vi "Canny Edge Detection.vi"(4 "Threshold 2":dbl=100.0, 6 "Threshold 1":dbl=50.0, 7 "Aperture Size":T1, 8 "error in (no error)":errorcluster, 10 "Canny Edge Result in":T2, 11 "Greyscale Image-Source in":T2) -> (0 "error out":errorcluster, 3 "Canny Edge":T2)   [LabVIEW 2020, in "image.lvlib"]
doc: "Apply the Canny Edge Detetction operation to the source image."
uses:
  image.lvlib
  Greyscale Image.ctl
  Canny Aperture Size.ctl
  common/common.lvlib
  common/bin/gartoolkit_32-1.dll
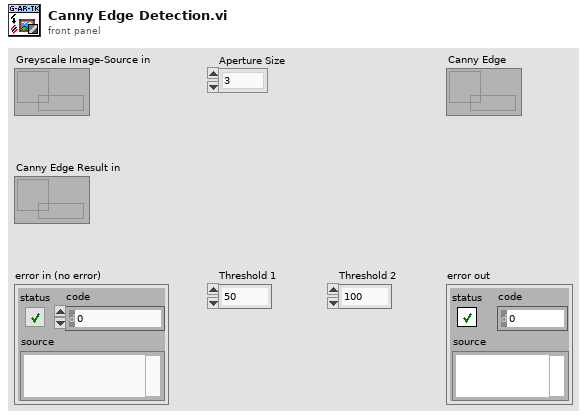
[diagram p1: front panel]
types:
  T1 = typedef "image.lvlib/Canny Aperture Size.ctl" = enum16{"3", "5", "7"}
  T2 = typedef "image.lvlib/Greyscale Image.ctl" = refnum<data-value>
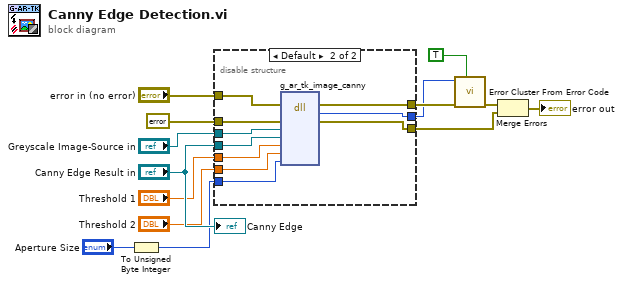
[diagram p0: block diagram]
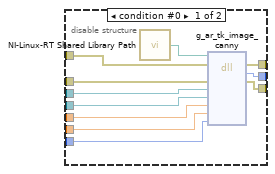
[diagram p2: hidden frame]
diagram:
  n1 = To Unsigned Byte Integer(number="Aperture Size") -> (unsigned 8bit integer=w5:u8)
  n2 = disable-structure shown="Default" {
    disable-tunnel: "error in (no error)" -> [w25 w35]
    disable-tunnel: errorcluster {"status"=FALSE, "code"=0, "source"=""} ("error constant") -> [w24 w34]
    disable-tunnel: "Greyscale Image-Source in" -> [w23 w33]
    disable-tunnel: "Canny Edge Result in" -> [w22 w32]
    disable-tunnel: "Threshold 1" -> [w21 w31]
    disable-tunnel: "Threshold 2" -> [w20 w30]
    disable-tunnel: w5 -> [w19 w29]
    disable-tunnel: [w18 w28] -> w4
    disable-tunnel: [w17 w27] -> w3
    disable-tunnel: [w16 w26] -> w2
    frame condition #0 {
      n3 = call "NI-Linux-RT Shared Library Path.vi"() -> ("Path"=w15:path)
      n4 = dll-call lib="?" fn="g_ar_tk_image_canny" ("g_ar_toolkit.*.*:g_ar_tk_image_in_range")(path in=w15, error in=w25, "error_cluster"=w24, "EDVR src"=w23, "EDVR dst"=w22, "threshold_1"=w21, "threshold_2"=w20, "aperture_size"=w19) -> (error out=w18:errorcluster, w17:i32, "error_cluster"=w16:errorcluster)  [unwired: 6 in, 1 out]
    }
    frame condition #1 (active) {
      n5 = dll-call lib="C:/serenial/lib/g-augmented-reality-toolkit/LabVIEW/common/bin/gartoolkit_*-1.*" fn="g_ar_tk_image_canny" ("g_ar_toolkit.*.*:g_ar_tk_image_in_range")(error in=w35, "error_cluster"=w34, "EDVR src"=w33, "EDVR dst"=w32, "threshold_1"=w31, "threshold_2"=w30, "aperture_size"=w29) -> (error out=w28:errorcluster, w27:i32, "error_cluster"=w26:errorcluster)  [unwired: 7 in, 1 out]
    }
  }
  n6 = call <vilib>:"Error Cluster From Error Code.vi"("show call chain? (False)"=TRUE, "error in (no error)"=w4, "error code (0)"=w3) -> ("error out"=w12:errorcluster)  [unwired: 6 in]
  n7 = Merge Errors(w12, w2) -> (→"error out":errorcluster)
  "Canny Edge" <- "Canny Edge Result in"
